vi "Create All Endpoints as Load.vi"(8 "error in":errorcluster, 9 "topology":string, 10 "switches json":string, 11 "endpoint configuration in":T1 format="%.0x") -> (0 "error out":errorcluster, 3 "endpoint configuration out":T1 format="%.0x")   [LabVIEW 2020, in "SLSC Switch Scripting.lvlib"]
uses:
  SLSC Switch Scripting.lvlib
  <vilib>/NI VeriStand/Custom Device API/Custom Device Item Ref.ctl
  Shared/Endpoint Configuration Cluster.ctl
  Shared/Endpoint Configuration Enum.ctl
  Dependencies.llb/SLSC Switch Shared.lvlib
  <vilib>/NI VeriStand/Custom Device API/Custom Device API.lvlib
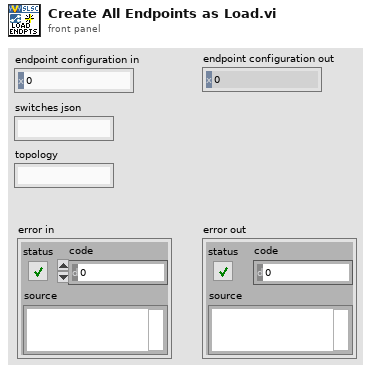
[diagram p1: front panel]
types:
  T1 = typedef "Custom Device API.lvlib/Custom Device Item Ref.ctl" = u64
  T2 = typedef "SLSC Switch Shared.lvlib/Endpoint Configuration Enum.ctl" = enum16{"Load", "Source", "Configuration"}
  T3 = typedef "SLSC Switch Shared.lvlib/Endpoint Configuration Cluster.ctl" = cluster{"Endpoint":string, "Configuration":T2}
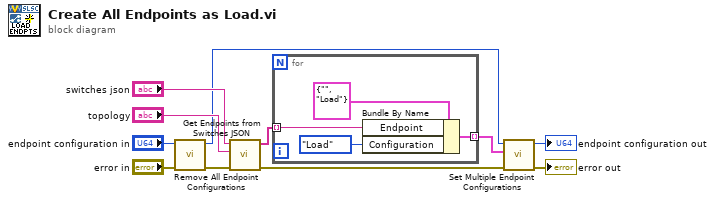
[diagram p0: block diagram]
diagram:
  n1 = call "Remove All Endpoint Configurations.vi"("error in"="error in", "endpoint configuration in"="endpoint configuration in") -> ("error out"=w4:errorcluster, "endpoint configuration out"=w1:T1)  [unwired: 8 in]
  n2 = call "Get Endpoints from Switches JSON.vi"("error in"=w4, "topology"="topology", "switches json"="switches json") -> ("error out"=w11:errorcluster, "endpoints"=w8:string[])  [unwired: 7 in]
  n3 = for {
    tunnel: w8 -> [w14] mode=indexing
    tunnel: [w12] -> w5 mode=indexing
    n4 = Bundle By Name(cluster=T3 {"Endpoint"="", "Configuration"=enum."Load"} ("All Endpoint Configurations"), "Endpoint"=w14, "Configuration"=Endpoint_Configuration_Enum."Load") -> (w12:T3)
  }
  n5 = call "Set Multiple Endpoint Configurations.vi"("error in"=w11, "endpoint configurations"=w5, "endpoint configuration in"=w1) -> ("error out"=→"error out":errorcluster, "endpoint configuration out"=→"endpoint configuration out":T1)  [unwired: 7 in]
